vi "Test_GetClassName.vi"() -> ()   [LabVIEW 2017, in "TestLibrary.lvlib"]
uses:
  TestLibrary.lvlib
  GSharpCls_class/GSharpCls.lvclass
panel:
  in  "NXG extended-ascii converted string":string="   \u00015\u000bTestLibrary\u000bInteractive\u000bTestLibrary\u000fGSharpCls.gtype           "
  in  "NXG byte array":i32[](array[numeric])
  out "2017 string":string
  in  "byte array":u8[](array[numeric])=[0, 0, 0, 1, 37, 17, 84, 101, 115, 116, 76, 105, 98, 114, 97, 114, 121, 46, 108, 118, 108, 105, 98, 17, 71, 83, 104, 97, 114, 112, 67, 108, 115, 46, 108, 118, 99, 108, 97, 115, 115, 0, 0, 0, 0, 0, 0, 0, 0, 0, 0, 0]
  out "error out":errorcluster
  out "class name":string
  out "full class name":string
  out "lvlib hierarchy":string[](array[string])
  out "reference out":refnum<class "GSharpCls.lvclass">
  # "GSharpCls"
  # "TestLibrary.lvlib:GSharpCls.lvclass"
  # "varför har vi med lvclass i full name?\nbehöver vi det?\nvad använder vi det till?\nskall vi ha med .gtype i namnet då?\nvarför är inte klassen med i hierarchy?"
  # "TestLibrary"
  # "är inte detta GetNamespace man vill göra?"
  # "denna funktion tar bara knotrolltypen, inte datatypen"
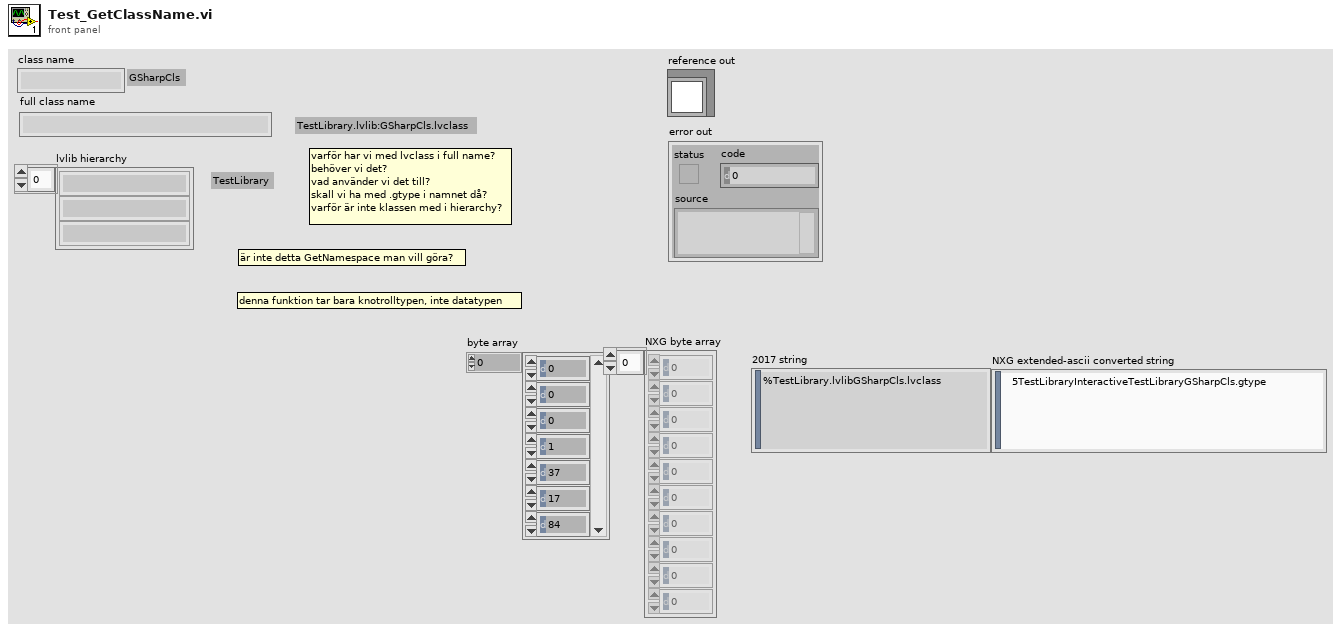
[diagram p1: front panel]
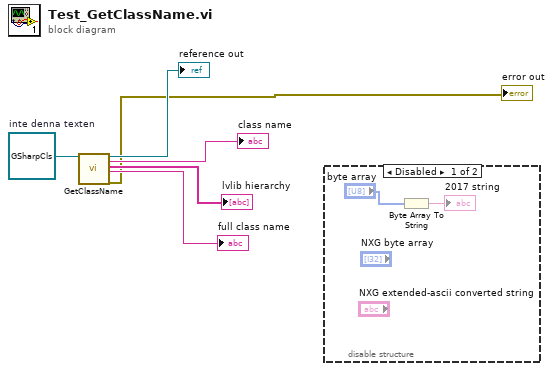
[diagram p0: block diagram]
diagram:
  w3 = refnum<class "GSharpCls.lvclass"> refnum  # inte denna texten
  n1 = call-dynamic "GetClassName.vi"("reference in"=w3) -> ("reference out"=→"reference out":refnum<class "GSharpCls.lvclass">, "class name"=→"class name":string, "lvlib hierarchy"=→"lvlib hierarchy":string[], "full class name"=→"full class name":string, "error out"=→"error out":errorcluster)  [unwired: 14 in]
  n2 = disable-structure shown="Disabled" {
    frame Disabled {
      n3 = Byte Array To String(unsigned byte array="byte array") -> (string=→"2017 string":string)
    }
    frame Enabled {
    }
  }
